vi "Convert filetype to Icon Image.vi"(8 "error in (no error)":errorcluster, 10 "is template?":bool, 11 "file type":T2) -> (0 "error out":errorcluster, 3 "image data":T1)   [LabVIEW 2020, in "NI_FileType.lvlib"]
doc: "Returns TRUE if this file type could be loaded with the Open VI Reference function. It includes VIs, Polymorphic VIs, Controls, Templates, and Globals."
uses:
  NI_FileType.lvlib
  FT_FileTypes.ctl
  imagedata.ctl
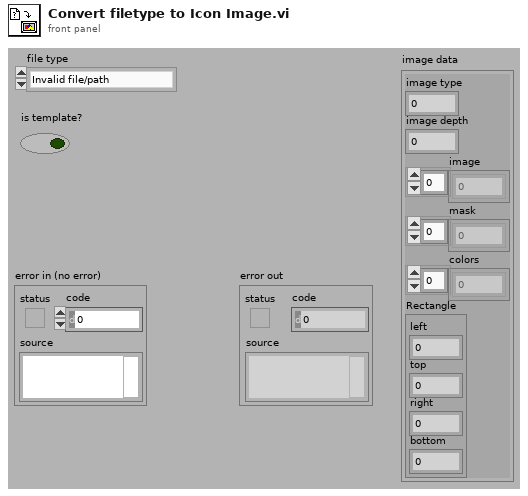
[diagram p1: front panel]
types:
  T1 = typedef "imagedata.ctl" = cluster{"image type":i32, "image depth":i32, "image":u8[], "mask":u8[], "colors":u32[], "Rectangle":cluster{"left":i16, "top":i16, "right":i16, "bottom":i16}}
  T2 = typedef "NI_FileType.lvlib/FT_FileTypes.ctl" = enum32{"Invalid file/path", "Unknown type", "Instrument", "Control", "Polymorphic VI", "Project", "Library", "LVClass", "XControl", "XNode", "CIN", "Run-time menu", "Palette menu", "LLB", "Shortcut", "Directory", "Class Private Data Control", "Statechart", "MathScript .m file", "Ladder Diagram", "LVLibp"}
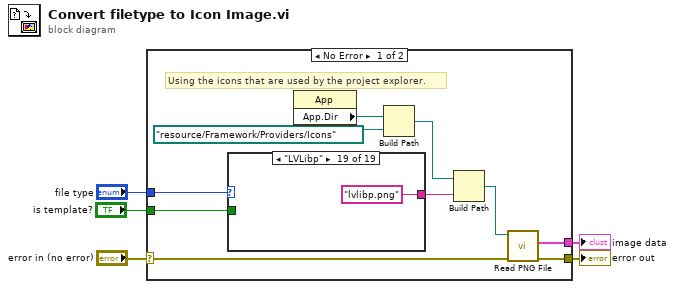
[diagram p0: block diagram]
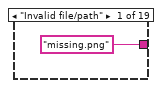
[diagram p2: hidden frame]
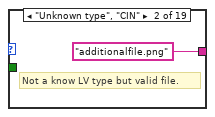
[diagram p3: hidden frame]
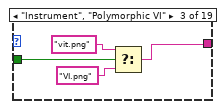
[diagram p4: hidden frame]
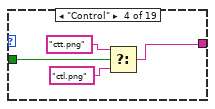
[diagram p5: hidden frame]
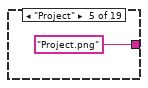
[diagram p6: hidden frame]
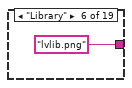
[diagram p7: hidden frame]
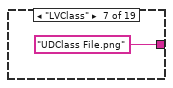
[diagram p8: hidden frame]
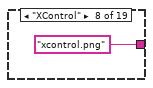
[diagram p9: hidden frame]
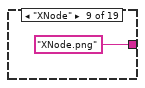
[diagram p10: hidden frame]
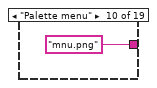
[diagram p11: hidden frame]
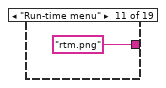
[diagram p12: hidden frame]
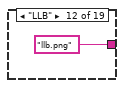
[diagram p13: hidden frame]
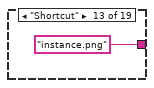
[diagram p14: hidden frame]
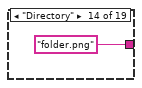
[diagram p15: hidden frame]
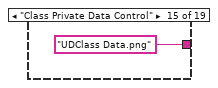
[diagram p16: hidden frame]
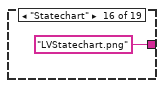
[diagram p17: hidden frame]
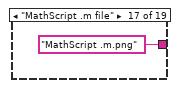
[diagram p18: hidden frame]
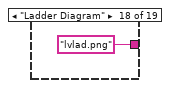
[diagram p19: hidden frame]
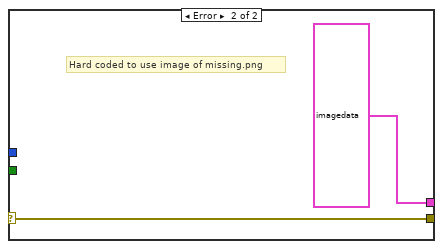
[diagram p20: hidden frame]
diagram:
  n1 = case shown="No Error" "error in (no error)" {
    selector: "error in (no error)" -> [w7 w42]
    tunnel: "file type" -> [w15 _]
    tunnel: [w9 T1 {"image type"=0, "image depth"=32, "image"=array[1024 elements], "mask"=[0, 0, 15, 224, 63, 248, 127, 252, 127, 252, 255, 254, 255, 254, 255, 254, 255, 254, 255, 254, 255, 254, 255, 254, 127, 252, 127, 252, 63, 248, 15, 224], "colors"=[], "Rectangle"={"left"=0, "top"=0, "right"=16, "bottom"=16}} ("image data")] -> w4
    tunnel: [w8 w42] -> w2
    tunnel: "is template?" -> [w6 _]
    frame No Error {
      # "Using the icons that are used by the project explorer."
      n2 = case shown="\"LVLibp\"" w15 {
        tunnel: ["missing.png" ("name or relative path") "additionalfile.png" ("name or relative path") w19 w22 "Project.png" ("name or relative path") "lvlib.png" ("name or relative path") "UDClass File.png" ("name or relative path") "xcontrol.png" ("name or relative path") "XNode.png" ("name or relative path") "mnu.png" ("name or relative path") "rtm.png" ("name or relative path") "llb.png" ("name or relative path") "instance.png" ("name or relative path") "folder.png" ("name or relative path") "UDClass Data.png" ("name or relative path") "LVStatechart.png" ("name or relative path") "MathScript .m.png" ("name or relative path") "lvlad.png" ("name or relative path") "lvlibp.png" ("name or relative path")] -> w10
        tunnel: w6 -> [_ _ w21 w23 _ _ _ _ _ _ _ _ _ _ _ _ _ _ _]
        frame "Invalid file/path" {
        }
        frame "Unknown type", "CIN" {
          # "Not a know LV type but valid file."
        }
        frame "Instrument", "Polymorphic VI" {
          n3 = Select(t="vit.png" ("name or relative path"), s=w21, f="VI.png" ("name or relative path")) -> (s? t:f=w19:string)
        }
        frame "Control" {
          n4 = Select(t="ctt.png" ("name or relative path"), s=w23, f="ctl.png" ("name or relative path")) -> (s? t:f=w22:string)
        }
        frame "Project" {
        }
        frame "Library" {
        }
        frame "LVClass" {
        }
        frame "XControl" {
        }
        frame "XNode" {
        }
        frame "Palette menu" {
        }
        frame "Run-time menu" {
        }
        frame "LLB" {
        }
        frame "Shortcut" {
        }
        frame "Directory" {
        }
        frame "Class Private Data Control" {
        }
        frame "Statechart" {
        }
        frame "MathScript .m file" {
        }
        frame "Ladder Diagram" {
        }
        frame "LVLibp" {
        }
      }
      n5 = property class="App"() -> ("App.Dir"=w14:path)  [unwired: 2 in, 2 out]
      n6 = Build Path(base path=w14, name or relative path=path "resource/Framework/Providers/Icons" ("Application:Directory Path")) -> (appended path=w12:path)
      n7 = Build Path(base path=w12, name or relative path=w10) -> (appended path=w11:path)
      n8 = call "Read PNG File.vi"("error in (no error)"=w7, "path to PNG file"=w11) -> ("error out"=w8:errorcluster, "image data"=w9:T1)  [unwired: 7 in, 1 out]
    }
    frame Error {
      # "Hard coded to use image of missing.png"
    }
  }
  "image data" <- w4
  "error out" <- w2
